vi "Inject Attribute List.vi"(6 "Attributes Ref":refnum<data-value>, 8 "error in (no error)":errorcluster, 11 "Start Pre-Soak in":refnum<class "Start Tire Shine Foam.lvclass">) -> (0 "error out":errorcluster, 3 "Start Pre-Soak out":refnum<class "Start Tire Shine Foam.lvclass">)   [LabVIEW 2019, in "Start Tire Shine Foam.lvclass"]
uses:
  <vilib>/gpm_packages/@cs/Car-wash/Source/Process Steps/Start Tire Shine Foam/Start Tire Shine Foam.lvclass
  <vilib>/gpm_packages/@cs/lookup-table/Source/LookupTable/LookupTable.lvclass
  <vilib>/gpm_packages/@cs/lookup-table/Source/LookupTable/LookupTable.lvclass/LookupTable.ctl
  <vilib>/gpm_packages/@cs/Car-wash/Source/Process Steps/Start Tire Shine Foam/Start Tire Shine Foam.lvclass/Start Tire Shine Foam.ctl
  49629b21-7cff-4f5c-8b74-717044878a8d.vi
  <vilib>/gpm_packages/@cs/lookup-table/Source/LookupTable/Read Table Reference.vi
  49629b21-7cff-4f5c-8b74-717044878a8d.vi/1c278cb4-125a-4332-a31a-d9f8fa4288d3.vi
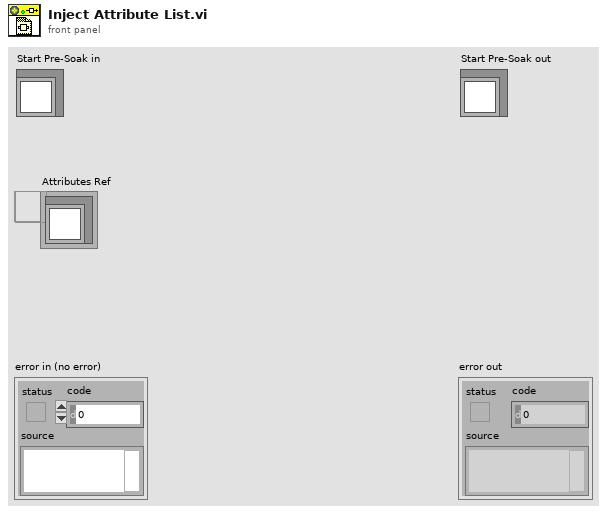
[diagram p1: front panel]
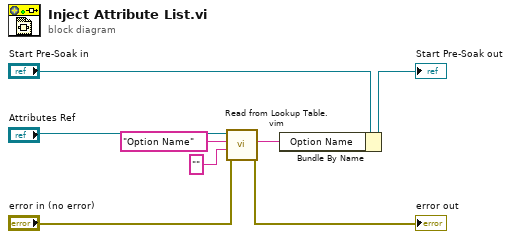
[diagram p0: block diagram]
diagram:
  n1 = call "Read from Lookup Table.vim"("error in (no error)"="error in (no error)", "Type"="", "Item Name"="Option Name", "LookupTable Reference"="Attributes Ref") -> ("error out"=→"error out":errorcluster, "Value"=w6:string)  [unwired: 4 in, 2 out]
  n2 = Bundle By Name(cluster="Start Pre-Soak in", "Option Name"=w6) -> (→"Start Pre-Soak out":refnum<class "Start Tire Shine Foam.lvclass">)
